vi "OnDataChange.vi"(0 "Microscope_RM21 in":refnum<class "Microscope_RM21.lvclass">, 1 "DataExchange":T1, 3 "error in (no error)":errorcluster) -> (7 "Microscope_RM21 out":refnum<class "Microscope_RM21.lvclass">, 10 "error out":errorcluster)   [LabVIEW 2020]
uses:
  Hardware Abstraction Layer/Component/Device/Device/DataExchange.ctl
  Interface/DataListener/DataListener.lvclass
  Microscope_RM21.lvclass
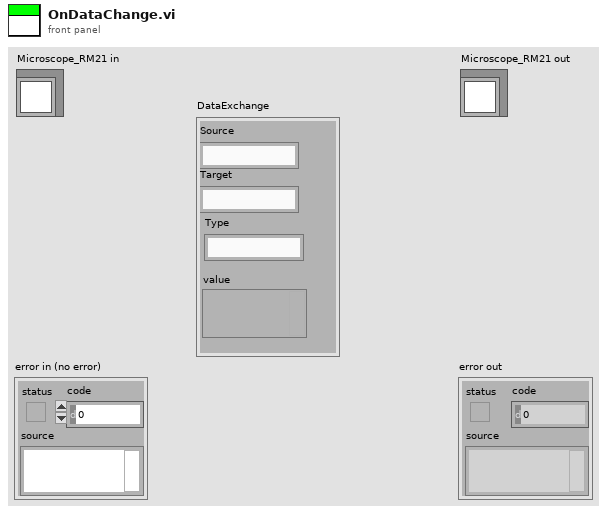
[diagram p1: front panel]
types:
  T1 = typedef "DataListener.lvclass/DataExchange.ctl" = cluster{"Source":string, "Target":string, "Type":string, "value":variant}
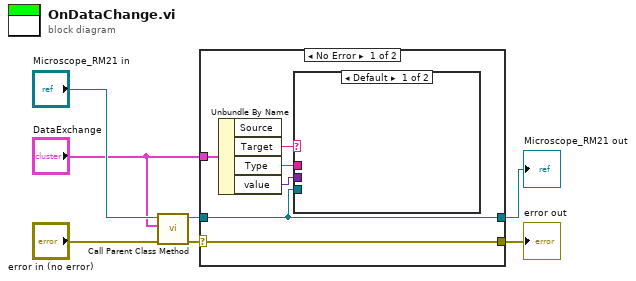
[diagram p0: block diagram]
diagram:
  n1 = call-parent "Call Parent Class Method"("Microscope in"="Microscope_RM21 in", "DataExchange"="DataExchange", "error in (no error)"="error in (no error)") -> ("Microscope out"=w3:refnum<class "Microscope_RM21.lvclass">, "error out"=w5:errorcluster)  [unwired: 6 in]
  n2 = case shown="No Error" w5 {
    selector: w5 -> [w13 w15]
    tunnel: [w13 w15] -> w1
    tunnel: [w8 w14] -> w2
    tunnel: w3 -> [w8 w14]
    tunnel: "DataExchange" -> [w12 _]
    frame No Error {
      n3 = Unbundle By Name(w12) -> ("Target"=w9:string, "Type"=w10:string, "value"=w11:variant)  [unwired: 1 out]
      n4 = case shown="Default" w9 {
        tunnel: w11 -> [_ _]
        tunnel: w10 -> [_ _]
        tunnel: w8 -> [_ _]
        frame Default {
        }
        frame "DeviceStatus1" {
        }
      }
    }
    frame Error {
    }
  }
  "error out" <- w1
  "Microscope_RM21 out" <- w2
